vi "init.vi"(8 "error in (no error)":errorcluster, 10 "xmlConfig":string, 11 "ILC in":refnum<class "ILC.lvclass">) -> (0 "error out":errorcluster, 3 "ILC out":refnum<class "ILC.lvclass">)   [LabVIEW 2013, in "ILCCommon.lvlib" / "ILC.lvclass"]
uses:
  <userlib>/Common/ILC/ILC/ILC.lvclass
  <userlib>/Common/ILC/Configuration/ILC.ctl
  <userlib>/Common/ILC/Configuration/InputChannels.ctl
  <userlib>/Common/ILC/Configuration/ScanRate_Hz_MultichannelOptions.ctl
  <userlib>/Common/SerialProtocols/Configuration/SerialConfig.ctl
  <userlib>/Common/SerialProtocols/Configuration/SerialProtocol.ctl
  <userlib>/Common/SerialProtocols/Configuration/ProtocolParameters.ctl
  <userlib>/Common/ILC/ILC/ILC.lvclass/ILC.ctl
  <userlib>/Common/ILC/Configuration/ILCConfiguration.lvlib
  <userlib>/Common/SerialProtocols/SerialProtocols.lvlib
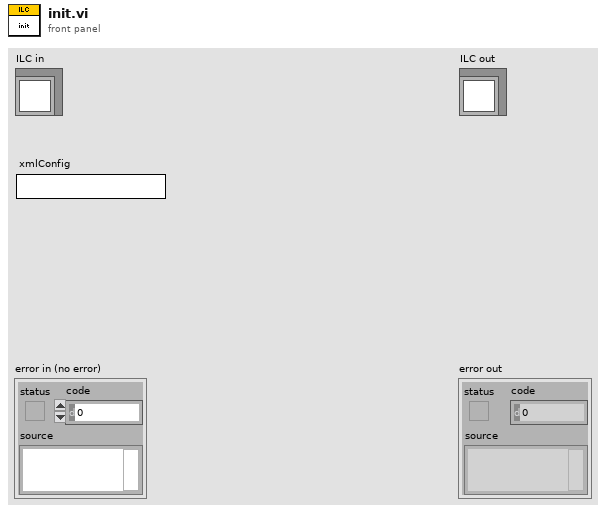
[diagram p1: front panel]
types:
  T1 = typedef "ILCCommon.lvlib/ILCConfiguration.lvlib/ILC.ctl" = cluster{"Input Channels":T2, "Scan Rate (Hz) ":T3, "ADC PGA Gain":u8, "SerialConfig":T4}
  T2 = typedef "ILCCommon.lvlib/ILCConfiguration.lvlib/InputChannels.ctl" = enum16{"Channel 0", "3 Channels", "5 Channels"}
  T3 = typedef "ILCCommon.lvlib/ILCConfiguration.lvlib/ScanRate_Hz_MultichannelOptions.ctl" = enum16{"50", "60", "100", "120", "200", "240", "300", "400", "480", "600", "1200", "2400", "4800"}
  T4 = typedef "SerialProtocols.lvlib/SerialConfig.ctl" = cluster{"Serial Protocol":T5, "Protocol Parameters":T6}
  T5 = typedef "SerialProtocols.lvlib/SerialProtocol.ctl" = enum16{"RS232", "RS485", "SerialSimulator"}
  T6 = typedef "SerialProtocols.lvlib/ProtocolParameters.ctl" = cluster{"VISA resource name":refnum<visa-resource-name>, "Baud Rate":u32, "Data Bits":u16, "Parity":enum16{"None", "Odd", "Even", "Mark", "Space"}, "Flow Control":u16, "Stop Bits":u16, "Timeout (ms)":u32}
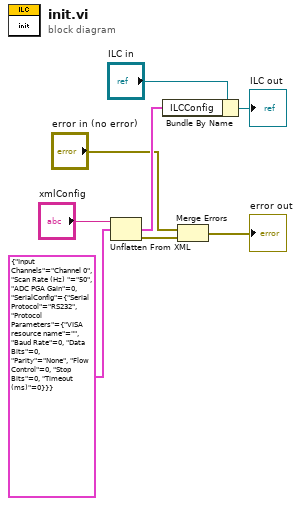
[diagram p0: block diagram]
diagram:
  n1 = Unflatten From XML(xml string="xmlConfig", type=T1 {"Input Channels"=enum."Channel 0", "Scan Rate (Hz) "=enum."50", "ADC PGA Gain"=0, "SerialConfig"={"Serial Protocol"=enum."RS232", "Protocol Parameters"={"VISA resource name"="", "Baud Rate"=0, "Data Bits"=0, "Parity"=enum."None", "Flow Control"=0, "Stop Bits"=0, "Timeout (ms)"=0}}} ("ILC")) -> (value=w6:T1, error out=w4:errorcluster)  [unwired: 1 in]
  n2 = Bundle By Name(cluster="ILC in", "ILCConfig"=w6) -> (→"ILC out":refnum<class "ILC.lvclass">)
  n3 = Merge Errors("error in (no error)", w4) -> (→"error out":errorcluster)
